vi "PCO_RecorderCreate.vi"(1 "wRecMode":u16(ring)=2 items=["PCO_RECORDER_MODE_FILE"=1, "PCO_RECORDER_MODE_MEMORY"=2, "PCO_RECORDER_MODE_CAMRAM"=3], 5 "phCamArr":u64[](array[numeric])=array[4097 elements], 7 "dwImgDistributionArr":u32[](array[numeric]), 9 "szDrive":path, 11 "error in (no error)":errorcluster {"code" format="%x"}) -> (4 "phRec out":u64, 6 "ErrorMessage":i32 format="%x", 8 "dwMaxImgCountArr":u32[](array[numeric]), 15 "error out":errorcluster {"code" format="%x"})   [LabVIEW 2020, in "Recorder.lvlib"]
doc: "<b>Description:</b>\nThis function creates the one and only instance of the recorder. It takes an array of handles to the required cameras as input parameter. If the function succeeds, those handles may not be used outside of the recorder until PCO_RecorderDelete is called. The main task of this function is to calculate the maximum recordable number of images for every camera by checking the available memory (RAM or Disk depending on the recorder mode) and the required distribution of the memory to the single cameras (e.g camera 1 should get twice as much available memory as camera 2, than the distribution would be [2, 1]). If the recorder is used in record to file mode, also the drive and the file type have to be specified, otherwise those parameters are just ignored.\nFunction will be rejected with error if a recorder was already created.\n\n<b>Note: </b>For file mode this function returns a warning, if the file name of the specified path already exists.\nThe function will be rejected with error if a recorder was already created.\n\n<b>Supported camera type:</b>\nAll cameras"
uses:
  Recorder.lvlib
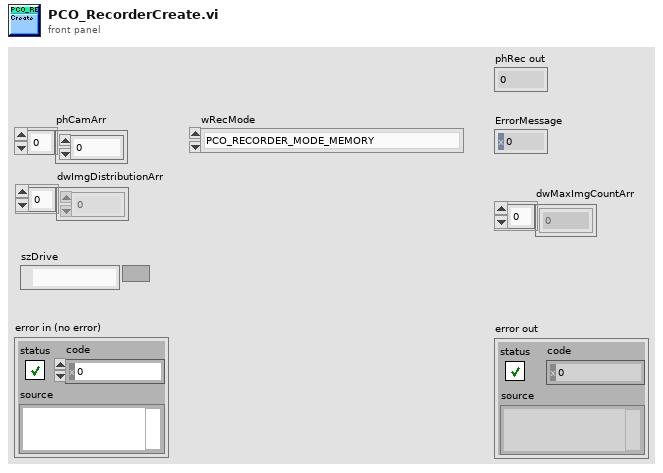
[diagram p1: front panel]
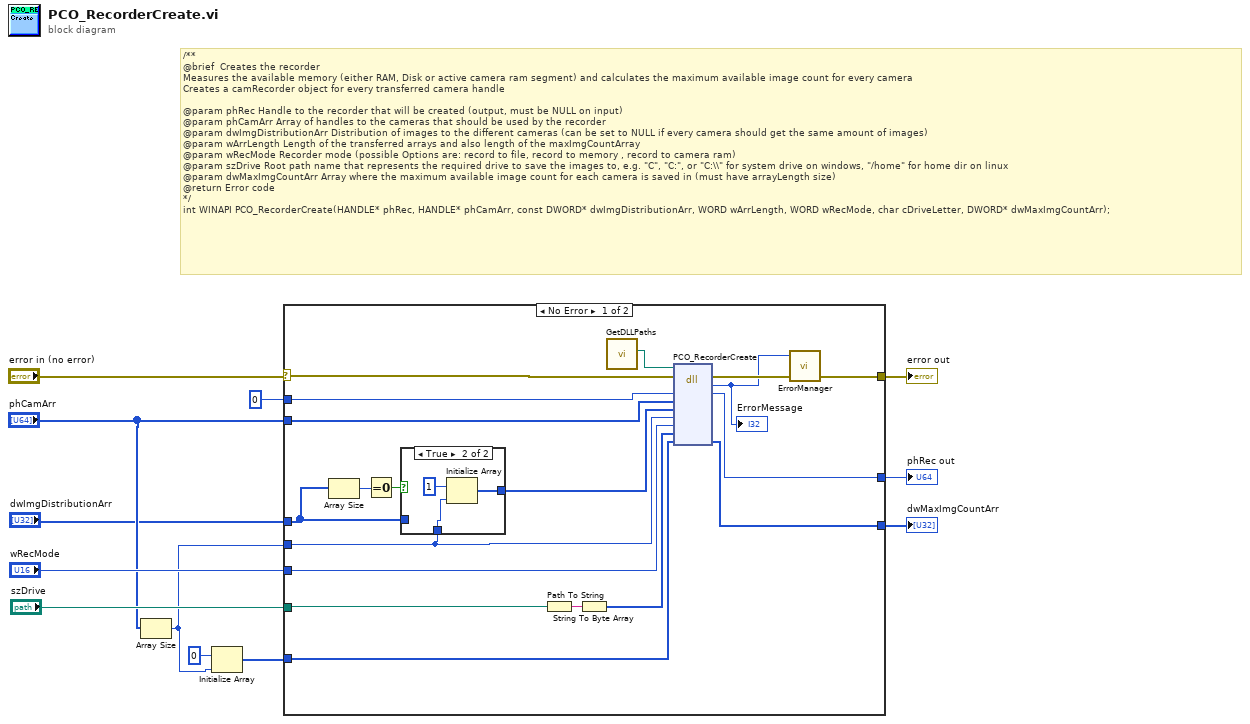
[diagram p0: block diagram]
diagram:
  # "/**\n@brief \tCreates the recorder\nMeasures the available memory (either RAM, Disk or active camera ram segment) and calculates the maximum available image count for every camera\nCreates a camRecorder object for every transferred camera handle\n\n@param phRec Handle to the recorder that will be created (output, must be NULL on input)\n@param phCamArr Array of handles to the cameras that should be used by the recorder\n@param dwImgDistributionArr Distribution of images to the different cameras (can be set to NULL if every camera should get the same amount of images)\n@param wArrLength Length of the transferred arrays and also length of the maxImgCountArray\n@param wRecMode Recorder mode (possible Options are: record to file, record to memory , record to camera ram)\n@param szDrive Root path name that represents the required drive to save the images to, e.g. \"C\", \"C:\", or \"C:\\\\\" for system drive on windows, \"/home\" for home dir on linux\n@param dwMaxImgCountArr Array where the maximum available image count for each camera is saved in (must have arrayLength size)\n@return Error code\n*/\nint WINAPI PCO_RecorderCreate(HANDLE* phRec, HANDLE* phCamArr, const DWORD* dwImgDistributionArr, WORD wArrLength, WORD wRecMode, char cDriveLetter, DWORD* dwMaxImgCountArr);"
  n1 = Array Size(array="phCamArr") -> (size(s)=w4:i32)
  n2 = Initialize Array(u32 0 ("element"), w4) -> (w5:u32[])
  n3 = case shown="No Error" "error in (no error)" {
    selector: "error in (no error)" -> [w26 w38]
    tunnel: u64 0 ("phRec") -> [w31 w37]
    tunnel: [w30 w37] -> w12
    tunnel: "phCamArr" -> [w23 _]
    tunnel: "dwImgDistributionArr" -> [w15 _]
    tunnel: "wRecMode" -> [w29 _]
    tunnel: [w28 w36] -> w10
    tunnel: [w25 w38] -> w9
    tunnel: "szDrive" -> [w27 _]
    tunnel: w5 -> [w24 w36]
    tunnel: w4 -> [w14 _]
    frame No Error {
      n4 = Array Size(array=w15) -> (size(s)=w17:i32)
      n5 = Equal To 0?(x=w17) -> (x = 0?=w16:bool)
      n6 = case shown="True" w16 {
        tunnel: w15 -> [w32 _]
        tunnel: w14 -> [_ w34]
        tunnel: [w32 w33] -> w13
        frame False {
        }
        frame True {
          n7 = Initialize Array(u32 1 ("element"), w34) -> (w33:u32[])
        }
      }
      n8 = Path To String(path=w27) -> (string=w22:string)
      n9 = String To Byte Array(string=w22) -> (unsigned byte array=w18:u8[])
      n10 = call "GetDLLPaths.vi"() -> ("PCO_Recorder_Path"=w19:path)  [unwired: 9 in, 2 out]
      n11 = dll-call lib="?" fn="PCO_RecorderCreate"(path in=w19, error in=w26, "phRec"=w31, "phCamArr"=w23, "dwImgDistributionArr"=w13, "wArrLength"=w14, "wRecMode"=w29, "szDrive"=w18, "dwMaxImgCountArr"=w24) -> (error out=w21:errorcluster, "return type"=w20:i32, "phRec"=w30:u64, "dwMaxImgCountArr"=w28:u32[])  [unwired: 6 in, 1 out]
      "ErrorMessage" <- w20
      n12 = call "ErrorManager.vi"("error in (no error)"=w21, "error code"=w20) -> ("error out"=w25:errorcluster)  [unwired: 3 in]
    }
    frame Error {
    }
  }
  "phRec out" <- w12
  "dwMaxImgCountArr" <- w10
  "error out" <- w9
